vi "test SSL Client Read Before Write.vi"(8 "error in (no error)":errorcluster, 11 "TestCase in":refnum<class "test SSL Client.lvclass">) -> (0 "error out":errorcluster, 3 "TestCase out":refnum<class "test SSL Client.lvclass">)   [LabVIEW 2013, in "test SSL Client.lvclass"]
uses:
  test SSL Client.lvclass
  NI OpenSSL Socket/SSL_Lib/SSL/SSL_Mode.ctl
  <vilib>/Utility/error.llb/DialogType.ctl
  suite SSL Client/suite SSL Client/SSL Context.vi
  <vilib>/addons/_JKI Toolkits/VI Tester/TestCase.llb/TestCase.lvclass
  NI OpenSSL Socket/SSL_Lib/BIO/BIO.lvclass
  NI OpenSSL Socket/SSL_Lib/SSL-Context/SSL-Context.lvclass
  NI OpenSSL Socket/SSL_Lib/SSL/SSL.lvclass
  suite SSL Client/suite SSL Client/suite SSL Client.lvclass
  NI OpenSSL Socket/SSL_Lib/SSL-Lib/SSL-Lib.lvclass
panel:
  out "x-y":u32
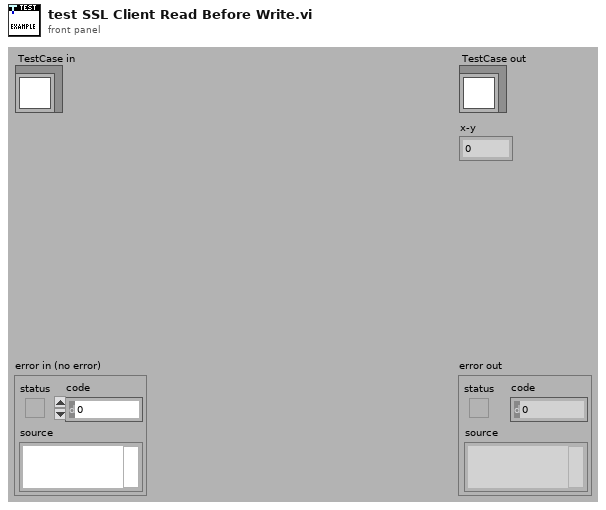
[diagram p1: front panel]
types:
  T1 = typedef "OpenSSL Socket.lvlib/SSL.lvclass/SSL_Mode.ctl" = i32
  T2 = typedef "DialogType.ctl" = u16
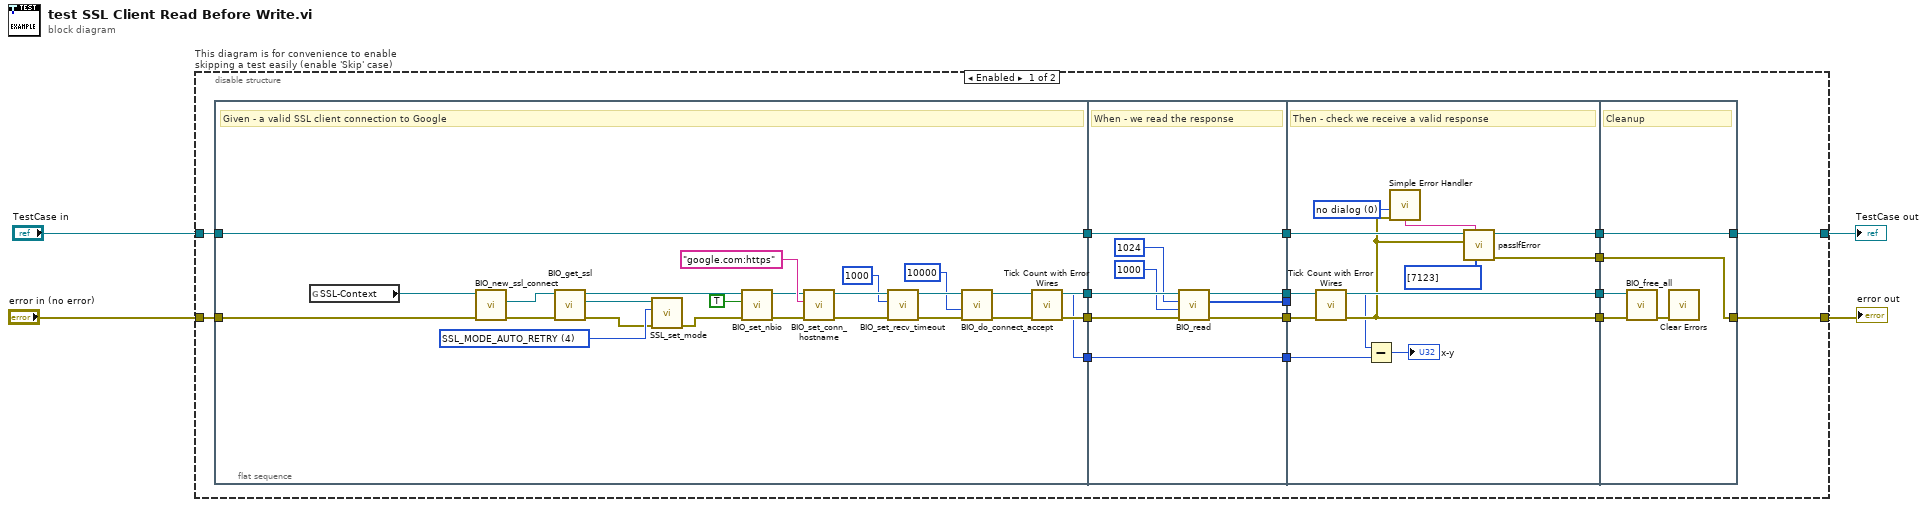
[diagram p0: block diagram]
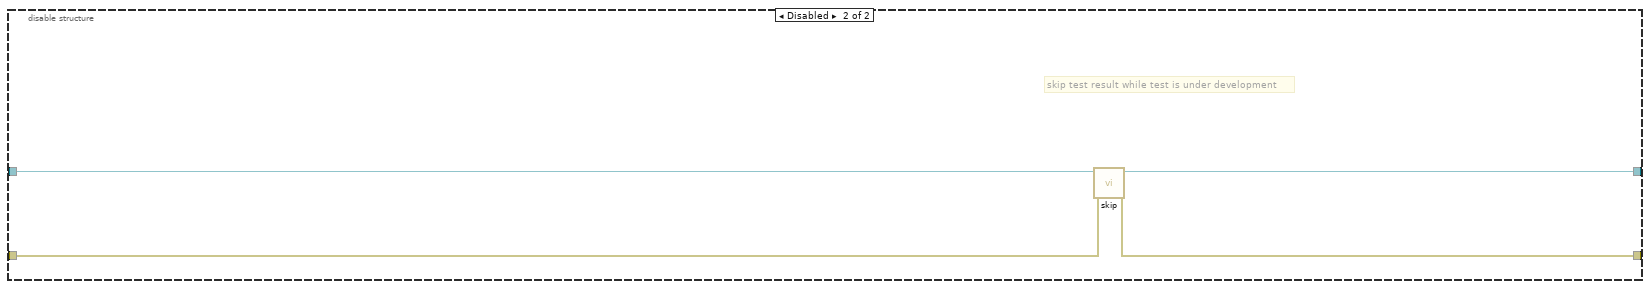
[diagram p2: hidden frame]
diagram:
  n1 = disable-structure "This diagram is for convenience to enable skipping a test easily (enable 'Skip' case)" shown="Enabled" {
    disable-tunnel: "TestCase in" -> [w16 w75]
    disable-tunnel: [w15 w73] -> w1
    disable-tunnel: [w14 w74] -> w3
    disable-tunnel: "error in (no error)" -> [w17 w72]
    frame Enabled {
      n2 = flat-sequence {
        tunnel: w17 -> [w38]
        tunnel: w16 -> [w37]
        tunnel: [w37] -> w21
        tunnel: [w29] -> w13
        tunnel: [w44] -> w12
        tunnel: [w28] -> w7
        tunnel: [w54] -> w20
        tunnel: [w51] -> w19
        tunnel: w21 -> [w54]
        tunnel: w13 -> [w53]
        tunnel: w12 -> [w52]
        tunnel: [w50] -> w11
        tunnel: [w49] -> w10
        tunnel: w7 -> [w48]
        tunnel: [w48] -> w6
        tunnel: [w65] -> w18
        tunnel: w20 -> [w66]
        tunnel: w19 -> [w61]
        tunnel: w11 -> [_]
        tunnel: w10 -> [w62]
        tunnel: [w62] -> w9
        tunnel: [w60] -> w8
        tunnel: w6 -> [w58]
        tunnel: [w55] -> w5
        tunnel: [w67] -> w14
        tunnel: [w71] -> w15
        tunnel: w18 -> [w71]
        tunnel: w9 -> [w69]
        tunnel: w8 -> [w70]
        tunnel: w5 -> [w67]
        frame #0 {
          w40 = T1 4 items=["None"=0, "SSL_MODE_ENABLE_PARTIAL_WRITE"=1, "SSL_MODE_ACCEPT_MOVING_WRITE_BUFFER"=2, "SSL_MODE_AUTO_RETRY"=4, "SSL_MODE_RELEASE_BUFFERS"=16, "SSL_MODE_SEND_FALLBACK_SCSV"=128] ("Mode")
          # "Given - a valid SSL client connection to Google"
          n3 = global read "SSL Context.vi" "SSL-Context"() -> (w36:refnum<class "SSL-Context.lvclass">)
          n4 = call "BIO_new_ssl_connect.vi"("error in (no error)"=w38, "SSL-Context in"=w36) -> ("error out"=w42:errorcluster, "BIO out"=w43:refnum<class "BIO.lvclass">)  [unwired: 7 in, 1 out]
          n5 = call "BIO_get_ssl.vi"("error in (no error)"=w42, "BIO in"=w43) -> ("error out"=w39:errorcluster, "SSL out"=w41:refnum<class "SSL.lvclass">, "BIO out"=w27:refnum<class "BIO.lvclass">)  [unwired: 7 in]
          n6 = call "SSL_set_mode.vi"("error in (no error)"=w39, "Mode"=w40, "SSL in"=w41) -> ("error out"=w25:errorcluster)  [unwired: 7 in, 1 out]
          n7 = call "BIO_set_nbio.vi"("error in (no error)"=w25, "Non-Blocking?"=TRUE, "BIO in"=w27) -> ("error out"=w24:errorcluster, "BIO out"=w26:refnum<class "BIO.lvclass">)  [unwired: 7 in]
          n8 = call "BIO_set_conn_hostname.vi"("error in (no error)"=w24, "Hostname"="google.com:https", "BIO in"=w26) -> ("error out"=w35:errorcluster, "BIO out"=w34:refnum<class "BIO.lvclass">)  [unwired: 7 in]
          n9 = call "BIO_set_recv_timeout.vi"("error in (no error)"=w35, "RECV timeout (ms)"=u32 1000, "BIO in"=w34) -> ("error out"=w32:errorcluster, "BIO out"=w33:refnum<class "BIO.lvclass">)  [unwired: 7 in]
          n10 = call "BIO_do_connect_accept.vi"("error in (no error)"=w32, "Timeout (10000ms)"=u32 10000, "BIO in"=w33) -> ("error out"=w30:errorcluster, "BIO out"=w44:refnum<class "BIO.lvclass">)  [unwired: 7 in]
          n11 = call "Tick Count with Error Wires.vi"("error in (no error)"=w30) -> ("error out"=w29:errorcluster, "millisecond timer value"=w28:u32)  [unwired: 9 in]
        }
        frame #1 {
          # "When - we read the response"
          n12 = call "BIO_read.vi"("error in (no error)"=w53, "Timeout (10000ms)"=u32 1000, "bytes to read"=1024, "BIO in"=w52) -> ("error out"=w51:errorcluster, "Bytes read"=w50:u8[], "BIO out"=w49:refnum<class "BIO.lvclass">)  [unwired: 5 in]
        }
        frame #2 {
          w63 = T2 0 items=["no dialog", "OK message", "continue or stop message", "OK message + warnings", "continue/stop + warnings"] ("type of dialog (OK msg:1)")
          # "Then - check we receive a valid response"
          n13 = call "Tick Count with Error Wires.vi"("error in (no error)"=w61) -> ("error out"=w60:errorcluster, "millisecond timer value"=w59:u32)  [unwired: 9 in]
          n14 = Subtract(x=w59, y=w58) -> (x-y=→"x-y":u32)
          n15 = call <vilib>:"Simple Error Handler.vi"("type of dialog (OK msg:1)"=w63, "error in (no error)"=w60) -> ("message"=w64:string)  [unwired: 3 in, 4 out]
          n16 = call-dynamic "passIfError.vi"("passing error codes (default = any error code)"=i32[] [7123], "custom report message (\"\")"=w64, "error"=w60, "TestCase in"=w66) -> ("error out"=w55:errorcluster, "TestCase out"=w65:refnum<class "test SSL Client.lvclass">)  [unwired: 6 in]
        }
        frame #3 {
          # "Cleanup"
          n17 = call "BIO_free_all.vi"("error in (no error)"=w70, "BIO in"=w69) -> ("error out"=w68:errorcluster)  [unwired: 9 in]
          n18 = call <vilib>:"Clear Errors.vi"("error in (no error)"=w68) -> ()  [unwired: 6 in, 1 out]
        }
      }
    }
    frame Disabled {
      # "skip test result while test is under development"
      n19 = call <vilib>:"skip.vi"("error in (no error)"=w72, "TestCase in"=w75) -> ("error out"=w74:errorcluster, "TestCase out"=w73:refnum<class "test SSL Client.lvclass">)  [unwired: 8 in]
    }
  }
  "error out" <- w3
  "TestCase out" <- w1
